vi "ADB-LMS_Esp32_Rst.vi"(11 "COM BLE Esp32":refnum<visa-resource-name>) -> (1 "Stat":bool, 2 "CMD Monitor":string="\r\n")   [LabVIEW 2018]
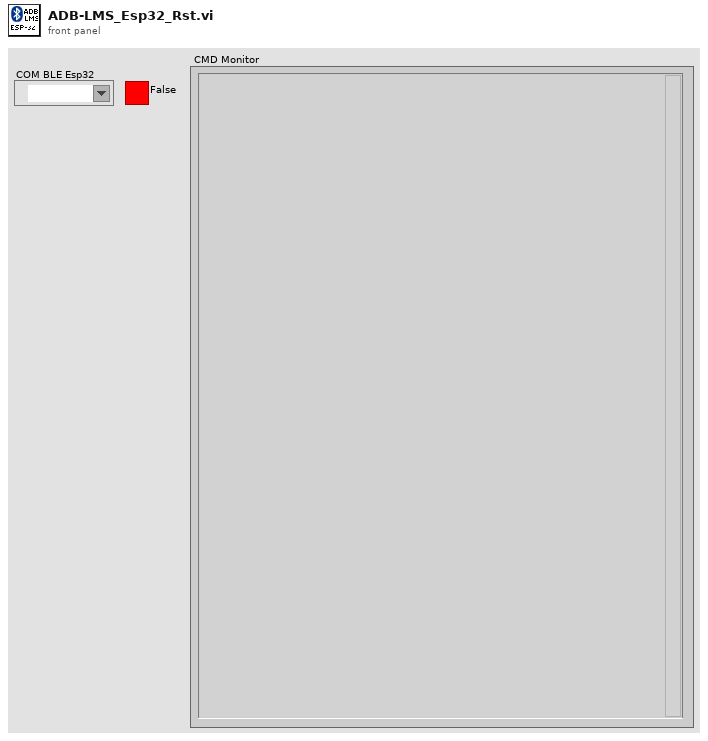
[diagram p1: front panel]
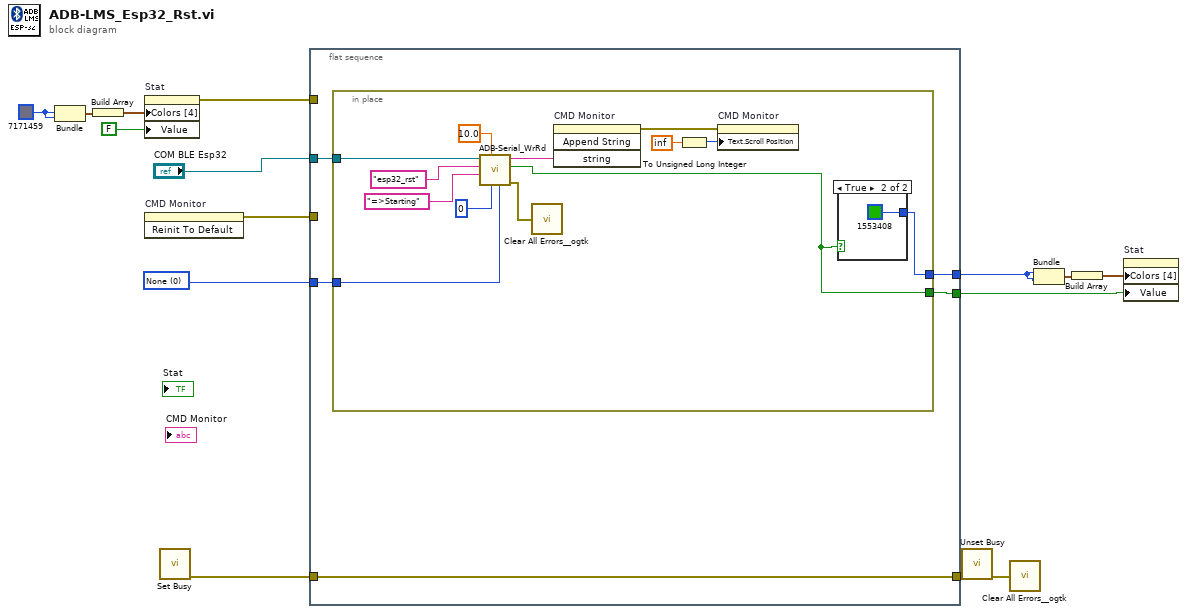
[diagram p0: block diagram]
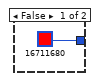
[diagram p2: hidden frame]
diagram:
  w14 = u32 7171459
  w3 = u16 0 items=["None", "XON/XOFF", "RTS/CTS", "XON/XOFF & RTS/CTS", "DTR/DSR", "XON/XOFF & DTR/DSR"] ("flow control (0:none)")
  n1 = Bundle(w14, w14) -> (w15:cluster{u32, u32})  [unwired: 1 in]
  n2 = Build Array(w15) -> (w12:cluster{u32, u32}[])
  n3 = property on="Stat" class="Bool (strict)"("Colors [4]"=w12, "Value"=FALSE ("Check  BLE")) -> (error out=w4:errorcluster)  [unwired: 2 in, 1 out]
  n4 = invoke on="CMD Monitor" class="Str" method="Reinit To Default"() -> (error out=w1:errorcluster)  [unwired: 3 in, 2 out]
  n5 = call <vilib>:"Set Busy.vi"() -> ("error out"=w13:errorcluster)  [unwired: 10 in, 1 out]
  n6 = flat-sequence {
    tunnel: [w20] -> w7
    tunnel: [w19] -> w6
    tunnel: [w18] -> w5
    tunnel: w13 -> [w20]
    tunnel: w4 -> [_]
    tunnel: w3 -> [w17]
    tunnel: "COM BLE Esp32" -> [w16]
    tunnel: w1 -> [_]
    frame #0 {
      n7 = in-place {
        in-place-border: w16 -> [w32]
        in-place-border: w17 -> [w25]
        in-place-border: [w21] -> w19
        in-place-border: [w22] -> w18
        n8 = call "ADB-Serial_WrRd.vi"("flow control (0:none)"=w25, "Tx Deay"=u16 0, "Timeout(Sec)"=10.0, "PassString"="=>Starting", "Command"="esp32_rst", "ComPort"=w32) -> ("error out"=w28:errorcluster, "PASS"=w22:bool, "received"=w23:string)  [unwired: 3 in]
        n9 = call <userlib>:"Clear All Errors__ogtk.vi"("Error In"=w28) -> ()  [unwired: 3 in, 1 out]
        n10 = invoke on="CMD Monitor" class="Str" method="Append String"("string"=w23) -> (error out=w24:errorcluster)  [unwired: 3 in, 3 out]
        n11 = To Unsigned Long Integer(number=inf) -> (unsigned 32bit integer=w26:u32)
        n12 = property on="CMD Monitor" class="Str"(error in=w24, "Text.Scroll Position"=w26) -> ()  [unwired: 1 in, 2 out]
        n13 = case shown="True" w22 {
          tunnel: [u32 16711680 u32 1553408] -> w21
          frame False {
          }
          frame True {
          }
        }
      }
    }
  }
  n14 = call <vilib>:"Unset Busy.vi"("error in (no error)"=w7) -> ("error out"=w8:errorcluster)  [unwired: 10 in]
  n15 = call <userlib>:"Clear All Errors__ogtk.vi"("Error In"=w8) -> ()  [unwired: 3 in, 1 out]
  n16 = Bundle(w6, w6) -> (w9:cluster{u32, u32})  [unwired: 1 in]
  n17 = Build Array(w9) -> (w10:cluster{u32, u32}[])
  n18 = property on="Stat" class="Bool (strict)"("Colors [4]"=w10, "Value"=w5) -> ()  [unwired: 2 in, 2 out]
